vi "Restore Default Setting.vi"(8 "error in (no error)":errorcluster, 11 "hdl in":i32) -> (0 "error out":errorcluster, 3 "hdl out":i32)   [LabVIEW 2011, in "Thorlabs_MDT69xB.lvlib"]
doc: "Restores default factory settings."
uses:
  <instrlib>/Thorlabs_MDT69xB/Thorlabs_MDT69xB.lvlib
  <instrlib>/Thorlabs_MDT69xB/Data/MDT_COMMAND_LIB_win32.dll
  <instrlib>/Thorlabs_MDT69xB/Data/MDT_COMMAND_LIB_x64.dll
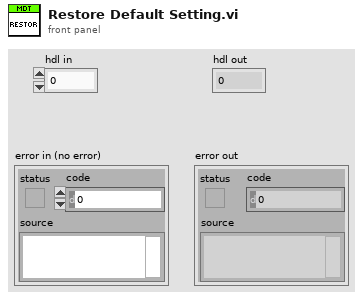
[diagram p1: front panel]
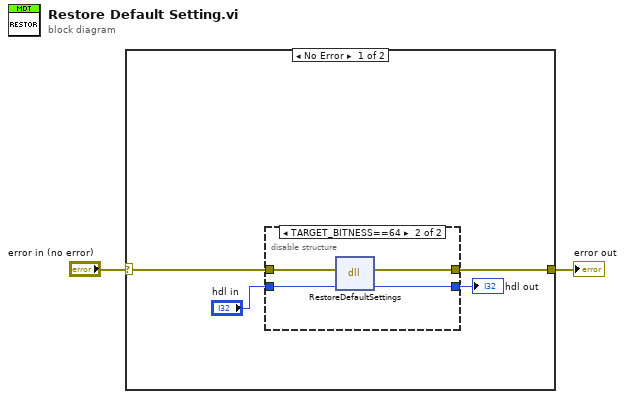
[diagram p0: block diagram]
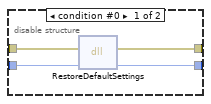
[diagram p2: hidden frame]
diagram:
  n1 = case shown="No Error" "error in (no error)" {
    selector: "error in (no error)" -> [w6 w15]
    tunnel: [w5 w15] -> w2
    frame No Error {
      n2 = disable-structure shown="TARGET_BITNESS==64" {
        disable-tunnel: w6 -> [w10 w14]
        disable-tunnel: [w9 w13] -> w5
        disable-tunnel: "hdl in" -> [w8 w12]
        disable-tunnel: [w7 w11] -> w3
        frame condition #0 {
          n3 = dll-call lib="E:/Program Files (x86)/National Instruments/LabVIEW 2011/instr.lib/Thorlabs_MDT69xB/Data/MDT_COMMAND_LIB_win32.dll" fn="RestoreDefaultSettings"(error in=w10, "hdl"=w8) -> (error out=w9:errorcluster, "hdl"=w7:i32)  [unwired: 3 in, 1 out]
        }
        frame condition #1 (active) {
          n4 = dll-call lib="C:/Program Files/National Instruments/LabVIEW 2011/instr.lib/Thorlabs_MDT69xB/Data/MDT_COMMAND_LIB_x64.dll" fn="RestoreDefaultSettings"(error in=w14, "hdl"=w12) -> (error out=w13:errorcluster, "hdl"=w11:i32)  [unwired: 3 in, 1 out]
        }
      }
      "hdl out" <- w3
    }
    frame Error {
    }
  }
  "error out" <- w2
